vi "OnlineAnalyzer.vi"() -> ()   [LabVIEW 2015]
uses:
  <vilib>/Analysis/3filter.llb/Filter Passband Type.ctl
  <vilib>/Analysis/2dsp.llb/Real FFT.vi
  <vilib>/Analysis/3filter.llb/Butterworth Filter (DBL).vi
  <vilib>/Analysis/NI_AALPro.lvlib
  <vilib>/Analysis/NI_AALBase.lvlib
panel:
  in  "FFT size":i32=-1
  in  "order":i32=2
  in  "low cutoff freq: fl":dbl=0.12500000000000006 format="%0.4f"
  in  "high cutoff freq: fh":dbl=0.45000000000000007 format="%0.2f"
  in  "sampling freq: fs":dbl=1.0 format="%0.2f"
  in  "filter type":T1
  out "Waveform Graph":dbl[][](graph)
  out "appended array":dbl[](array[numeric])
  in  "stop":bool
  out "size(s)":i32
  out "Waveform Graph 2":dbl[][](graph)
  out "AccVal":dbl
  out "x-y":i32
  out "number":i32
  out "YLDRMPortOut":refnum<visa-resource-name>
  in  "YLDRMPortInp":refnum<visa-resource-name>
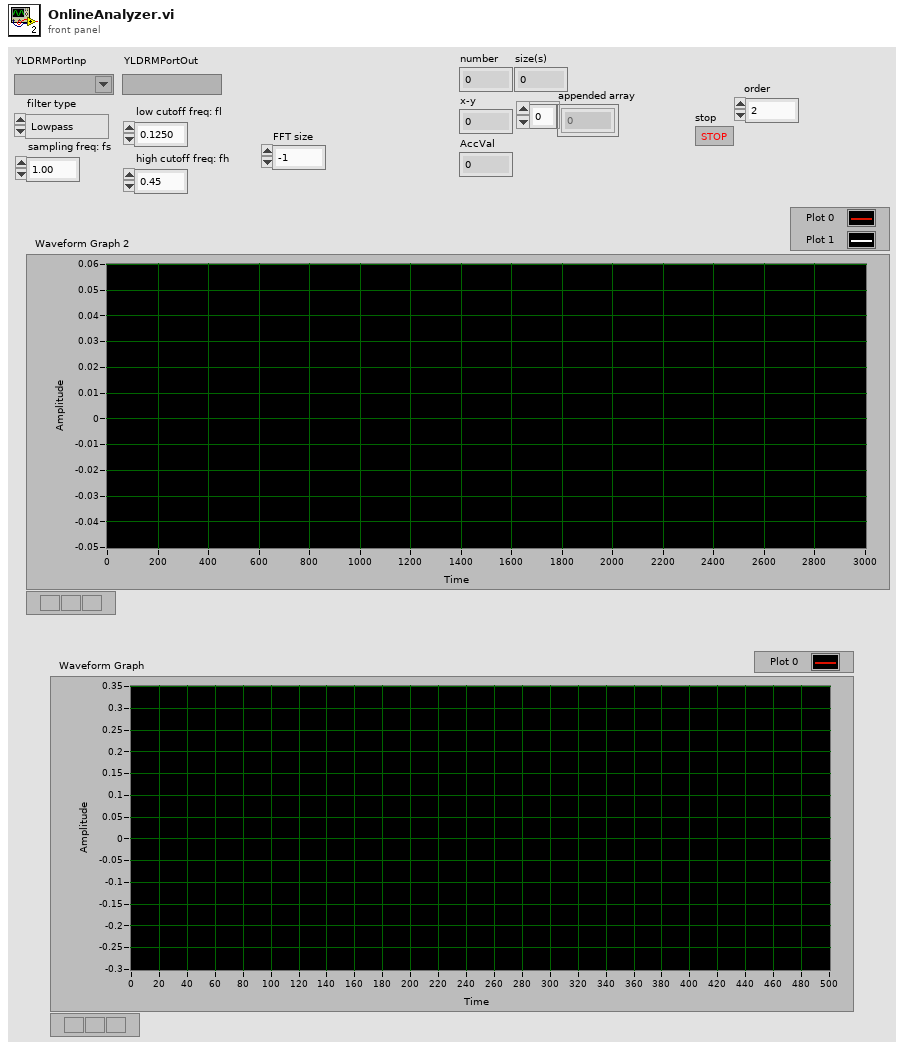
[diagram p1: front panel]
types:
  T1 = typedef "NI_AALBase.lvlib/Filter Passband Type.ctl" = enum32{"Lowpass", "Highpass", "Bandpass", "Bandstop"}
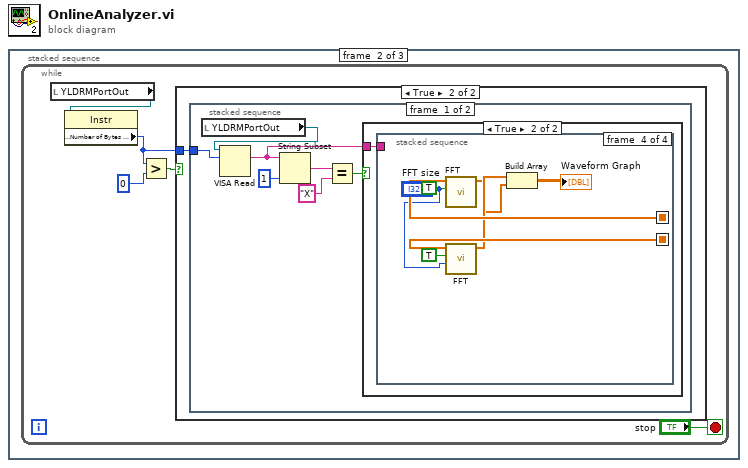
[diagram p0: block diagram]
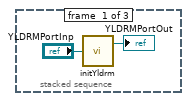
[diagram p2: hidden frame]
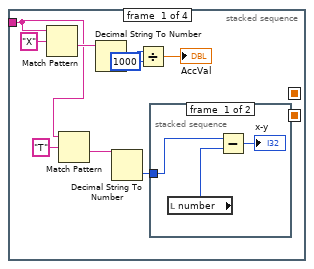
[diagram p5: hidden frame]
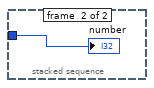
[diagram p6: hidden frame]
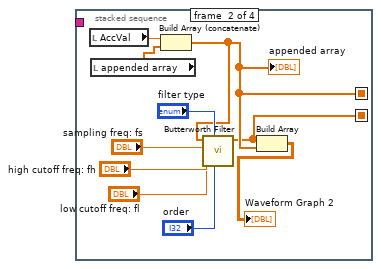
[diagram p7: hidden frame]
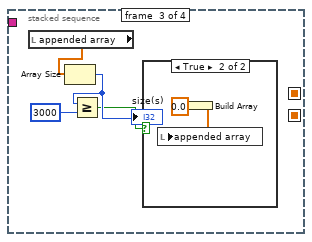
[diagram p8: hidden frame]
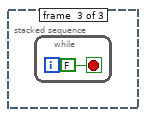
[diagram p11: hidden frame]
diagram:
  n1 = stacked-sequence {
    frame #0 {
      n2 = call "initYldrm.vi"("YLDRMPortInp"="YLDRMPortInp") -> ("YLDRMPortOut"=→"YLDRMPortOut":refnum<visa-resource-name>)  [unwired: 1 out]
    }
    frame #1 {
      n3 = while {
        stop <- "stop" stop-if-true
        n4 = local read "YLDRMPortOut"() -> (w7:refnum<visa-resource-name>)
        n5 = property class="Instr"(reference=w7) -> ("Serial Settings:Number of Bytes at Serial Port"=w4:u32)  [unwired: 1 in, 2 out]
        n6 = Greater?(x=w4, y=u32 0) -> (0:w5:bool)
        n7 = case shown="True" w5 {
          tunnel: w4 -> [_ w8]
          frame False {
          }
          frame True {
            n8 = stacked-sequence {
              tunnel: w8 -> [w14 _]
              frame #0 {
                n9 = local read "YLDRMPortOut"() -> (w15:refnum<visa-resource-name>)
                n10 = VISA Read(VISA resource name=w15, byte count=w14) -> (read buffer=w9:string)  [unwired: 1 in, 3 out]
                n11 = String Subset(string=w9, length (rest)=1 ("length (rest)")) -> (substring=w12:string)  [unwired: 1 in]
                n12 = Equal?(x=w12, y="X") -> (x = y?=w10:bool)
                n13 = case shown="True" w10 {
                  tunnel: w9 -> [_ w16]
                  frame False {
                  }
                  frame True {
                    n14 = stacked-sequence {
                      seq-local: [_ w31 _ _] -> [_ _ _ w53]
                      seq-local: [_ w30 _ _] -> [_ _ _ w52]
                      tunnel: w16 -> [w22 _ _ _]
                      frame #0 {
                        n15 = Match Pattern(string=w22, regular expression="X") -> (after substring=w24:string)  [unwired: 1 in, 3 out]
                        n16 = Match Pattern(string=w22, regular expression="T") -> (after substring=w21:string)  [unwired: 1 in, 3 out]
                        n17 = Decimal String To Number(string=w24) -> (number=w19:i32)  [unwired: 2 in, 1 out]
                        n18 = Decimal String To Number(string=w21) -> (number=w20:i32)  [unwired: 2 in, 1 out]
                        n19 = Divide(x=w19, y=1000) -> (x/y=→"AccVal":dbl)
                        n20 = stacked-sequence {
                          tunnel: w20 -> [w28 w29]
                          frame #0 {
                            n21 = local read "number"() -> (w27:i32)
                            n22 = Subtract(x=w28, y=w27) -> (x-y=→"x-y":i32)
                          }
                          frame #1 {
                            "number" <- w29
                          }
                        }
                      }
                      frame #1 {
                        n23 = local read "AccVal"() -> (w39:dbl)
                        n24 = local read "appended array"() -> (w37:dbl[])
                        n25 = Build Array (concatenate)(w39, w37) -> (w31:dbl[])
                        "appended array" <- w31
                        n26 = call-poly <vilib>:"Butterworth Filter.vi"("order"="order", "filter type"="filter type", "low cutoff freq: fl"="low cutoff freq: fl", "high cutoff freq: fh"="high cutoff freq: fh", "sampling freq: fs"="sampling freq: fs", "X"=w31) -> ("Filtered X"=w30:dbl[])  [unwired: 2 in, 1 out]
                        n27 = Build Array(w30, w31) -> (→"Waveform Graph 2":dbl[][])
                      }
                      frame #2 {
                        n28 = local read "appended array"() -> (w43:dbl[])
                        n29 = Array Size(array=w43) -> (size(s)=w42:i32)
                        "size(s)" <- w42
                        n30 = Greater Or Equal?(x=w42, y=3000) -> (x >= y?=w40:bool)
                        n31 = case shown="True" w40 {
                          frame False {
                          }
                          frame True {
                            n32 = Build Array(0.0) -> (w44:dbl[])
                            n33 = local write "appended array"(w44) -> ()
                          }
                        }
                      }
                      frame #3 {
                        n34 = call-poly <vilib>:"FFT.vi"("FFT size"="FFT size", "shift?"=TRUE, "X"=w53) -> ("FFT {X}"=w48:cdb[])  [unwired: 7 in, 1 out]
                        n35 = call-poly <vilib>:"FFT.vi"("FFT size"="FFT size", "shift?"=TRUE, "X"=w52) -> ("FFT {X}"=w49:cdb[])  [unwired: 7 in, 1 out]
                        n36 = Build Array(w49, w48) -> (→"Waveform Graph":cdb[][])
                      }
                    }
                  }
                }
              }
              frame #1 {
              }
            }
          }
        }
      }
    }
    frame #2 {
      n37 = while {
        stop <- FALSE stop-if-true
      }
    }
  }
